vi "Memory.vi"(11 "memory":u8[](array[numeric])) -> (3 "output cluster":T1)   [LabVIEW 2015, in "Igor.lvclass"]
uses:
  Igor.lvclass
  Memory.ctl
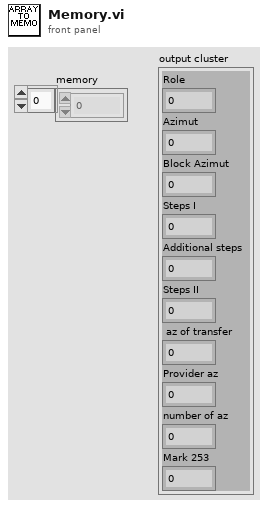
[diagram p1: front panel]
types:
  T1 = typedef "Memory.ctl" = cluster{"Role":i32, "Azimut":i32, "Block Azimut":i32, "Steps I":u32, "Additional steps":i32, "Steps II":u32, " az of transfer":u32, "Provider az":u32, "number of az":u32, "Mark 253":u32}
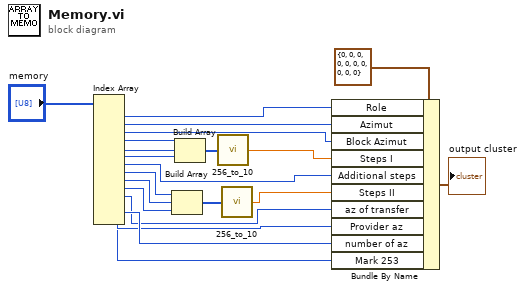
[diagram p0: block diagram]
diagram:
  n1 = Index Array(array="memory") -> (element #1=w4:u8, element #2=w5:u8, element #3=w8:u8, element #4=w9:u8, element #5=w7:u8, element #6=w6:u8, element #7=w12:u8, element #8=w13:u8, element #9=w14:u8, element #10=w15:u8, element #11=w18:u8, element #12=w19:u8, element #13=w20:u8, element #14=w1:u8)  [unwired: 14 in]
  n2 = Build Array(w13, w14, w15) -> (w16:u8[])
  n3 = Build Array(w9, w7, w6) -> (w10:u8[])
  n4 = call "256_to_10.vi"("Array"=w10) -> ("Numeric"=w11:dbl)
  n5 = call "256_to_10.vi"("Array"=w16) -> ("Numeric"=w17:dbl)
  n6 = Bundle By Name(cluster=T1 {"Role"=0, "Azimut"=0, "Block Azimut"=0, "Steps I"=0, "Additional steps"=0, "Steps II"=0, " az of transfer"=0, "Provider az"=0, "number of az"=0, "Mark 253"=0}, "Role"=w4, "Azimut"=w5, "Block Azimut"=w8, "Steps I"=w11, "Additional steps"=w12, "Steps II"=w17, "az of transfer"=w18, "Provider az"=w19, "number of az"=w20, "Mark 253"=w1) -> (→"output cluster":T1)
